vi "测量数据区_正常.vi"(11 "数组":u16[](array[numeric]) format="%04xH") -> (3 "测量数据区":T1 {"单位" items=["ug/L", "mg/L", "ppm", "mg/m3", "cm", "ppb", "ug/m3", "%", "nmol/mol", "umol/mol", "MPN/L", "MPN/100ml", "ng/m3", "NTU", "无量纲", "ms/cm", "us/cm", "℃", "mV", "万个/L"]})   [LabVIEW 2016, in "斯坦道总磷总氮.lvlib"]
uses:
  <vilib>/Utility/miscctls.llb/LVDateTimeRec.ctl
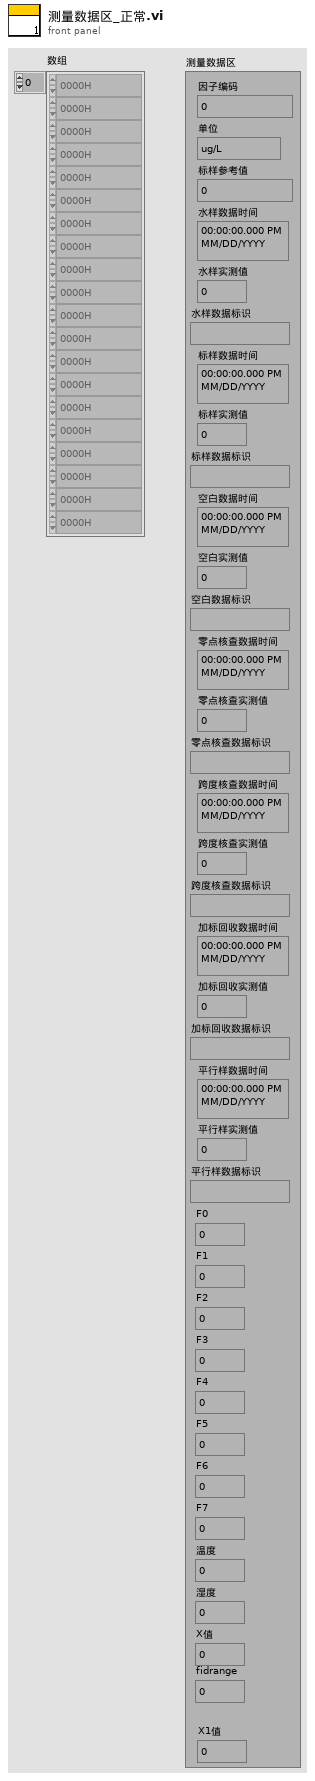
[diagram p1: front panel]
types:
  T1 = cluster{"因子编码":u32, "单位":u16, "标样参考值":sgl, "水样数据时间":timestamp, "水样实测值":sgl, "水样数据标识":string, "标样数据时间":timestamp, "标样实测值":sgl, "标样数据标识":string, "空白数据时间":timestamp, "空白实测值":sgl, "空白数据标识":string, "零点核查数据时间":timestamp, "零点核查实测值":sgl, "零点核查数据标识":string, "跨度核查数据时间":timestamp, "跨度核查实测值":sgl, "跨度核查数据标识":string, "加标回收数据时间":timestamp, "加标回收实测值":sgl, "加标回收数据标识":string, "平行样数据时间":timestamp, "平行样实测值":sgl, "平行样数据标识":string, "F0":sgl, "F1":sgl, "F2":sgl, "F3":sgl, "F4":sgl, "F5":sgl, "F6":sgl, "F7":sgl, "温度":sgl, "湿度":sgl, "X值":sgl, "fidrange":u16, "X1值":sgl}
  T2 = typedef "LVDateTimeRec.ctl" = cluster{"fractional second":dbl, "second":i32, "minute":i32, "hour":i32, "day of month":i32, "month":i32, "year":i32, "day of week":i32, "day of year":i32, "DST":i32}
  T3 = cluster{u32, u16, sgl, "time stamp":timestamp, sgl, string, "time stamp":timestamp, sgl, string, "time stamp":timestamp, sgl, string, "time stamp":timestamp, sgl, string, "time stamp":timestamp, sgl, string, "time stamp":timestamp, sgl, string, "time stamp":timestamp, sgl, string, sgl, sgl, sgl, sgl, sgl, sgl, sgl, sgl, sgl, sgl, sgl, "数值":u16, sgl}
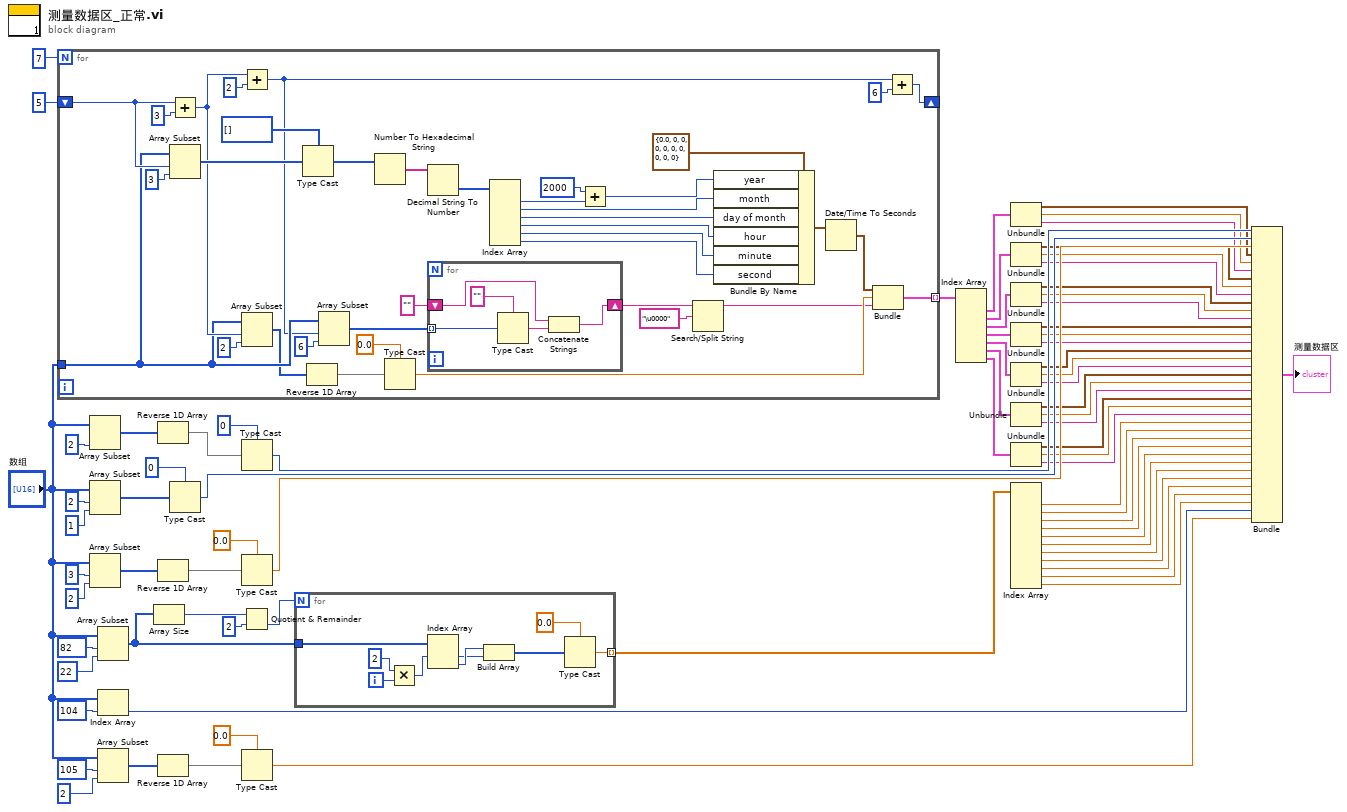
[diagram p0: block diagram]
diagram:
  n1 = for {
    N: 7 -> [_]
    tunnel: "数组" -> [w89]
    shift-right: [w78] -> _
    shift-left: 5 ("索引") -> [w96]
    tunnel: [w81] -> w41 mode=indexing
    n2 = Add(x=w96, y=3) -> (x+y=w92:i32)
    n3 = Array Subset(array=w89, index=w96, length=3 ("索引")) -> (w102:u16[])
    n4 = Add(x=w92, y=2) -> (x+y=w80:i32)
    n5 = Array Subset(array=w89, index=w92, length=2 ("长度")) -> (w77:u16[])
    n6 = Type Cast(type=u8[] [], x=w102) -> (*(type *) &x=w104:u8[])
    n7 = Reverse 1D Array(array=w77) -> (reversed array=w76:u16[])
    n8 = Array Subset(array=w89, index=w80, length=6 ("长度")) -> (w85:u16[])
    n9 = Number To Hexadecimal String(2:w104) -> (0:w103:string[])  [unwired: 1 in]
    n10 = Type Cast(type=sgl 0.0, x=w76) -> (*(type *) &x=w83:sgl)
    n11 = Decimal String To Number(string=w103) -> (number=w101:i32[])  [unwired: 2 in, 1 out]
    n12 = for {
      shift-right: [w117] -> w87
      shift-left: "" -> [w114]
      tunnel: w85 -> [w116] mode=indexing
      n13 = Type Cast(type="", x=w116) -> (*(type *) &x=w113:string)
      n14 = Concatenate Strings(w114, w113) -> (w117:string)
    }
    n15 = Index Array(array=w101) -> (element #1=w99:i32, element #2=w109:i32, element #3=w108:i32, element #4=w107:i32, element #5=w106:i32, element #6=w97:i32)  [unwired: 6 in]
    n16 = Add(x=2000 ("y"), y=w99) -> (x+y=w98:i32)
    n17 = Search/Split String(string=w87, search string/char (-)="\u0000" ("搜索字符串")) -> (substring before match=w82:string)  [unwired: 1 in, 2 out]
    n18 = Bundle By Name(cluster=T2 {"fractional second"=0.0, "second"=0, "minute"=0, "hour"=0, "day of month"=0, "month"=0, "year"=0, "day of week"=0, "day of year"=0, "DST"=0} ("日期时间记录"), "year"=w98, "month"=w109, "day of month"=w108, "hour"=w107, "minute"=w106, "second"=w97) -> (w105:T2)
    n19 = Date/Time To Seconds(2:w105) -> (0:w84:timestamp)  [unwired: 1 in]
    n20 = Bundle("time stamp"=w84, w83, w82) -> (w81:cluster{"time stamp":timestamp, sgl, string})  [unwired: 1 in]
    n21 = Add(x=w80, y=6) -> (x+y=w78:i32)
  }
  n22 = Array Subset(array="数组", length=u32 2 ("长度")) -> (w10:u16[])  [unwired: 1 in]
  n23 = Array Subset(array="数组", index=2 ("索引"), length=1 ("长度")) -> (w52:u16[])
  n24 = Array Subset(array="数组", index=3 ("索引"), length=2 ("长度")) -> (w9:u16[])
  n25 = Array Subset(array="数组", index=82 ("索引"), length=22 ("长度")) -> (w7:u16[])
  n26 = Index Array(array="数组", index=104 ("索引")) -> (element=w57:u16)
  n27 = Array Subset(array="数组", index=105 ("索引"), length=2 ("长度")) -> (w2:u16[])
  n28 = Array Size(array=w7) -> (size(s)=w6:i32)
  n29 = Reverse 1D Array(array=w10) -> (reversed array=w11:u16[])
  n30 = Reverse 1D Array(array=w9) -> (reversed array=w8:u16[])
  n31 = Reverse 1D Array(array=w2) -> (reversed array=w1:u16[])
  n32 = Type Cast(type=u16 0, x=w52) -> (*(type *) &x=w51:u16)
  n33 = Type Cast(type=u32 0, x=w11) -> (*(type *) &x=w54:u32)
  n34 = Type Cast(type=sgl 0.0, x=w8) -> (*(type *) &x=w46:sgl)
  n35 = Quotient & Remainder(x=w6, y=2) -> (floor(x/y)=w4:i32)  [unwired: 1 out]
  n36 = Type Cast(type=sgl 0.0, x=w1) -> (*(type *) &x=w42:sgl)
  n37 = for {
    N: w4 -> [_]
    tunnel: w7 -> [w126]
    tunnel: [w118] -> w3 mode=indexing
    i -> [w125]
    n38 = Multiply(x=2, y=w125) -> (x*y=w123:i32)
    n39 = Index Array(array=w126, index #1=w123) -> (element #1=w121:u16, element #2=w122:u16)  [unwired: 1 in]
    n40 = Build Array(w122, w121) -> (w120:u16[])
    n41 = Type Cast(type=sgl 0.0, x=w120) -> (*(type *) &x=w118:sgl)
  }
  n42 = Index Array(array=w41) -> (element #1=w40:cluster{"time stamp":timestamp, sgl, string}, element #2=w39:cluster{"time stamp":timestamp, sgl, string}, element #3=w38:cluster{"time stamp":timestamp, sgl, string}, element #4=w37:cluster{"time stamp":timestamp, sgl, string}, element #5=w36:cluster{"time stamp":timestamp, sgl, string}, element #6=w35:cluster{"time stamp":timestamp, sgl, string}, element #7=w34:cluster{"time stamp":timestamp, sgl, string})  [unwired: 7 in]
  n43 = Unbundle(w40) -> ("time stamp"=w33:timestamp, w32:sgl, w31:string)
  n44 = Unbundle(w39) -> ("time stamp"=w30:timestamp, w29:sgl, w28:string)
  n45 = Unbundle(w38) -> ("time stamp"=w27:timestamp, w26:sgl, w25:string)
  n46 = Unbundle(w37) -> ("time stamp"=w24:timestamp, w23:sgl, w22:string)
  n47 = Unbundle(w36) -> ("time stamp"=w21:timestamp, w20:sgl, w19:string)
  n48 = Unbundle(w35) -> ("time stamp"=w18:timestamp, w17:sgl, w16:string)
  n49 = Unbundle(w34) -> ("time stamp"=w15:timestamp, w14:sgl, w13:string)
  n50 = Index Array(array=w3) -> (element #1=w69:sgl, element #2=w68:sgl, element #3=w67:sgl, element #4=w66:sgl, element #5=w65:sgl, element #6=w64:sgl, element #7=w63:sgl, element #8=w62:sgl, element #9=w61:sgl, element #10=w60:sgl, element #11=w59:sgl)  [unwired: 11 in]
  n51 = Bundle(w54, w51, w46, "time stamp"=w33, w32, w31, "time stamp"=w30, w29, w28, "time stamp"=w27, w26, w25, "time stamp"=w24, w23, w22, "time stamp"=w21, w20, w19, "time stamp"=w18, w17, w16, "time stamp"=w15, w14, w13, w69, w68, w67, w66, w65, w64, w63, w62, w61, w60, w59, "数值"=w57, w42) -> (→"测量数据区":T3)  [unwired: 1 in]
